vi "DuplicateWorkflows.vi"(8 "error in (no error)":errorcluster, 11 "Repo / Workspace Folder Path":path) -> (0 "error out":errorcluster)   [LabVIEW 2019, in "Hawkeye.lvlib"]
uses:
  Hawkeye.lvlib
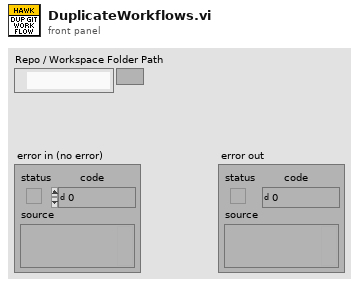
[diagram p1: front panel]
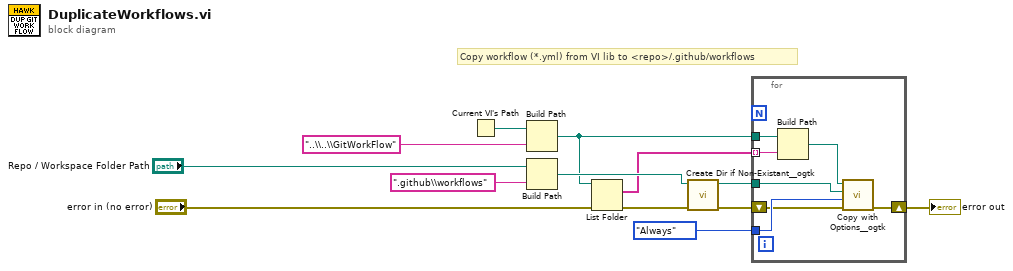
[diagram p0: block diagram]
diagram:
  # "Copy workflow (*.yml) from VI lib to <repo>/.github/workflows"
  n1 = Current VI's Path() -> (path=w1:path)
  n2 = Build Path(base path=w1, name or relative path="..\\..\\GitWorkFlow") -> (appended path=w5:path)
  n3 = Build Path(base path="Repo / Workspace Folder Path", name or relative path=".github\\workflows") -> (appended path=w8:path)
  n4 = List Folder(path=w5, error in="error in (no error)") -> (filenames=w4:string[], error out=w3:errorcluster)  [unwired: 2 in, 2 out]
  n5 = call <userlib>:"Create Dir if Non-Existant__ogtk.vi"("error in (no error)"=w3, "Directory Path"=w8) -> ("error out"=w6:errorcluster, "dup Directory Path"=w7:path)  [unwired: 7 in, 1 out]
  n6 = for {
    tunnel: enum16{"Never", "Always", "If Newer"}."Always" ("Replace Mode (Never)") -> [w20]
    tunnel: w7 -> [w18]
    shift-right: [w19] -> w13
    shift-left: w6 -> [w17]
    tunnel: w5 -> [w16]
    tunnel: w4 -> [w15] mode=indexing
    n7 = Build Path(base path=w16, name or relative path=w15) -> (appended path=w14:path)
    n8 = call <userlib>:"Copy with Options__ogtk.vi"("error in (no error)"=w17, "Replace Mode (Never)"=w20, "target path"=w18, "source path"=w14) -> ("error out"=w19:errorcluster)  [unwired: 6 in, 1 out]
  }
  "error out" <- w13
